vi "QA (子VI).vi"(0 "ori":dbl[][](array[numeric]), 1 "rec":dbl[][](array[numeric])) -> (2 "MSE_new":dbl, 3 "MSE":dbl, 4 "PSNR":dbl, 5 "SNR":dbl)   [LabVIEW 2018]
uses:
  <vilib>/Analysis/baseanly.llb/Mean (DBL).vi
  <vilib>/Analysis/NI_AALBase.lvlib
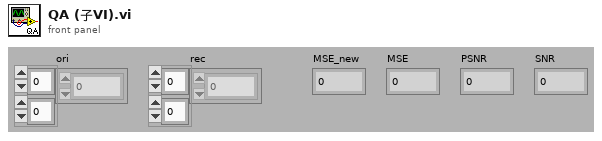
[diagram p1: front panel]
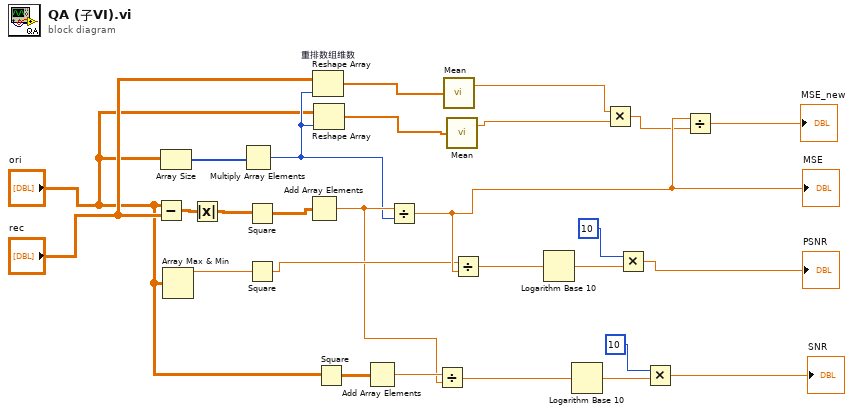
[diagram p0: block diagram]
diagram:
  n1 = Subtract(x="ori", y="rec") -> (x-y=w20:dbl[][])
  n2 = Array Size(array="ori") -> (size(s)=w17:i32[])
  n3 = Array Max & Min(array="ori") -> (max value=w16:dbl)  [unwired: 3 out]
  n4 = Absolute Value(x=w20) -> (abs(x)=w19:dbl[][])
  n5 = Multiply Array Elements(1:w17) -> (0:w6:i32)
  n6 = Square(x=w19) -> (x^2=w21:dbl[][])
  n7 = Square(x=w16) -> (x^2=w18:dbl)
  n8 = Add Array Elements(numeric array=w21) -> (sum=w9:dbl)
  n9 = Reshape Array "重排数组维数"("rec", w6) -> (w27:dbl[])
  n10 = Reshape Array("ori", w6) -> (w26:dbl[])
  n11 = Square(x="ori") -> (x^2=w11:dbl[][])
  n12 = Add Array Elements(numeric array=w11) -> (sum=w10:dbl)
  n13 = Divide(x=w9, y=w6) -> (x/y=w24:dbl)
  "MSE" <- w24
  n14 = Divide(x=w10, y=w9) -> (x/y=w2:dbl)
  n15 = call-poly <vilib>:"Mean.vi"("X"=w27) -> ("mean"=w8:dbl)  [unwired: 1 out]
  n16 = call-poly <vilib>:"Mean.vi"("X"=w26) -> ("mean"=w7:dbl)  [unwired: 1 out]
  n17 = Divide(x=w18, y=w24) -> (x/y=w15:dbl)
  n18 = Logarithm Base 10(1:w15) -> (0:w14:dbl)
  n19 = Logarithm Base 10(1:w2) -> (0:w3:dbl)
  n20 = Multiply(x=w8, y=w7) -> (x*y=w23:dbl)
  n21 = Multiply(x=u8 10, y=w14) -> (x*y=→"PSNR":dbl)
  n22 = Multiply(x=u8 10, y=w3) -> (x*y=→"SNR":dbl)
  n23 = Divide(x=w24, y=w23) -> (x/y=→"MSE_new":dbl)
